vi "RecordingControl_GetState.vi"(8 "Fehler (Eingang, kein Fehler)":errorcluster caption="Error_In", 11 "OXYGEN Ref In":refnum<visa-resource-name>) -> (0 "Fehler (Ausgang)":errorcluster caption="Error_Out", 1 "communication_data":T2, 2 "State":T1, 3 "OXYGEN Ref Out":refnum<visa-resource-name>)   [LabVIEW 2018, in "OXYGEN.lvlib"]
doc: "Queries the state of the recording operation {Started|Stopped|Stopping|Paused|Armed}."
uses:
  OXYGEN.lvlib
  TypeDefs/Cluster_RawCommData.ctl
  TypeDefs/RecordingControl_States.ctl
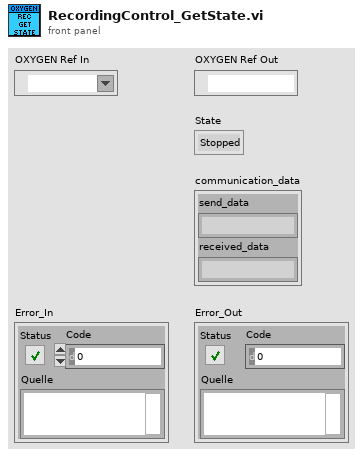
[diagram p1: front panel]
types:
  T1 = typedef "OXYGEN.lvlib/RecordingControl_States.ctl" = enum16{"Stopped", "Stopping", "Paused", "Started", "Armed"}
  T2 = typedef "OXYGEN.lvlib/Cluster_RawCommData.ctl" = cluster{"send_data":string, "received_data":string}
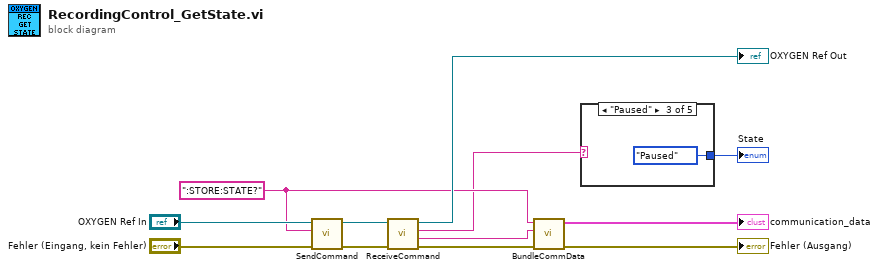
[diagram p0: block diagram]
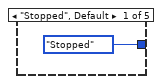
[diagram p2: hidden frame]
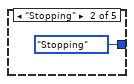
[diagram p3: hidden frame]
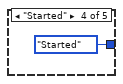
[diagram p4: hidden frame]
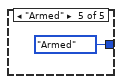
[diagram p5: hidden frame]
diagram:
  w7 = ":STORE:STATE?" ("Schreibpuffer")
  n1 = call "SendCommand.vi"("error in (no error)"="Fehler (Eingang, kein Fehler)", "String to Send"=w7, "OXY_SCPI Reseource In"="OXYGEN Ref In") -> ("error out"=w9:errorcluster, "OXY_SCPI Reseource Out"=w8:refnum<visa-resource-name>)  [unwired: 7 in]
  n2 = call "ReceiveCommand.vi"("error in (no error)"=w9, "OXY_SCPI Reseource In"=w8) -> ("error out"=w5:errorcluster, "received Data with Header"=w3:string, "received Data"=w2:string, "OXY_SCPI Reseource Out"=→"OXYGEN Ref Out":refnum<visa-resource-name>)  [unwired: 6 in]
  n3 = call "BundleCommData.vi"("error in (no error)"=w5, "received_data"=w3, "send_data"=w7) -> ("error out"=→"Fehler (Ausgang)":errorcluster, "communication_data"=→"communication_data":T2)  [unwired: 7 in]
  n4 = case shown="\"Paused\"" w2 {
    tunnel: [RecordingControl_States."Stopped" RecordingControl_States."Stopping" RecordingControl_States."Paused" RecordingControl_States."Started" RecordingControl_States."Armed"] -> w1
    frame "Stopped", Default {
    }
    frame "Stopping" {
    }
    frame "Paused" {
    }
    frame "Started" {
    }
    frame "Armed" {
    }
  }
  "State" <- w1
